vi "调阀对中 对中偏振角度.vi"(9 "角度":dbl[](array[numeric]), 10 "油压":dbl[](array[numeric]), 11 "扭矩":dbl[](array[numeric])) -> (1 "偏差角度":dbl, 3 "偏差扭矩":dbl format="%0.2f")   [LabVIEW 2015, in "Logging.lvlib"]
uses:
  Logging.lvlib
  <vilib>/Analysis/1siggen.llb/Ramp Pattern by Samples.vi
  <vilib>/Analysis/baseanly.llb/Mean (DBL).vi
  <vilib>/gmath/NI_Gmath.lvlib
  <vilib>/Analysis/NI_AALBase.lvlib
panel:
  out "角度反转回":dbl[](array[numeric])
  out "角度反转去":dbl[](array[numeric])
  out "角度正转回":dbl[](array[numeric])
  out "角度正转去":dbl[](array[numeric])
  out "油压反转回":dbl[](array[numeric])
  out "油压反转去":dbl[](array[numeric])
  out "油压正转回":dbl[](array[numeric])
  out "油压正转去":dbl[](array[numeric])
  out "扭矩反转回":dbl[](array[numeric])
  out "扭矩反转去":dbl[](array[numeric])
  out "扭矩正转回":dbl[](array[numeric])
  out "扭矩正转去":dbl[](array[numeric])
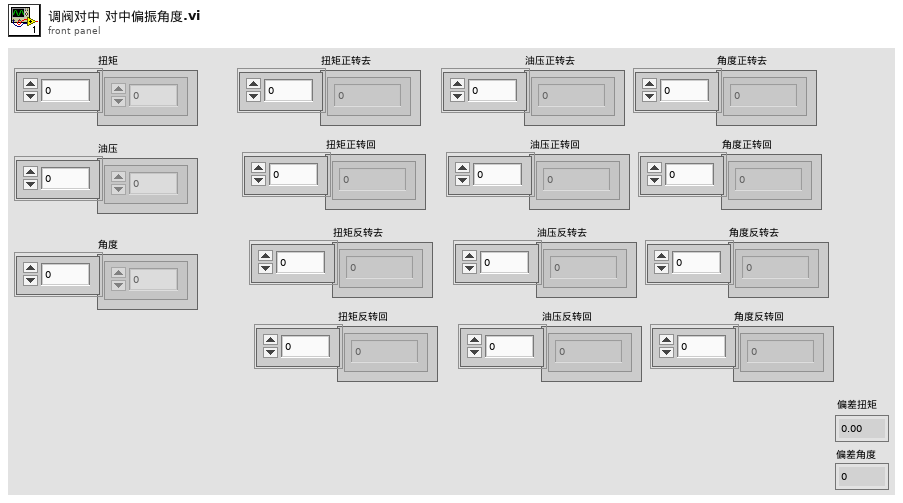
[diagram p1: front panel]
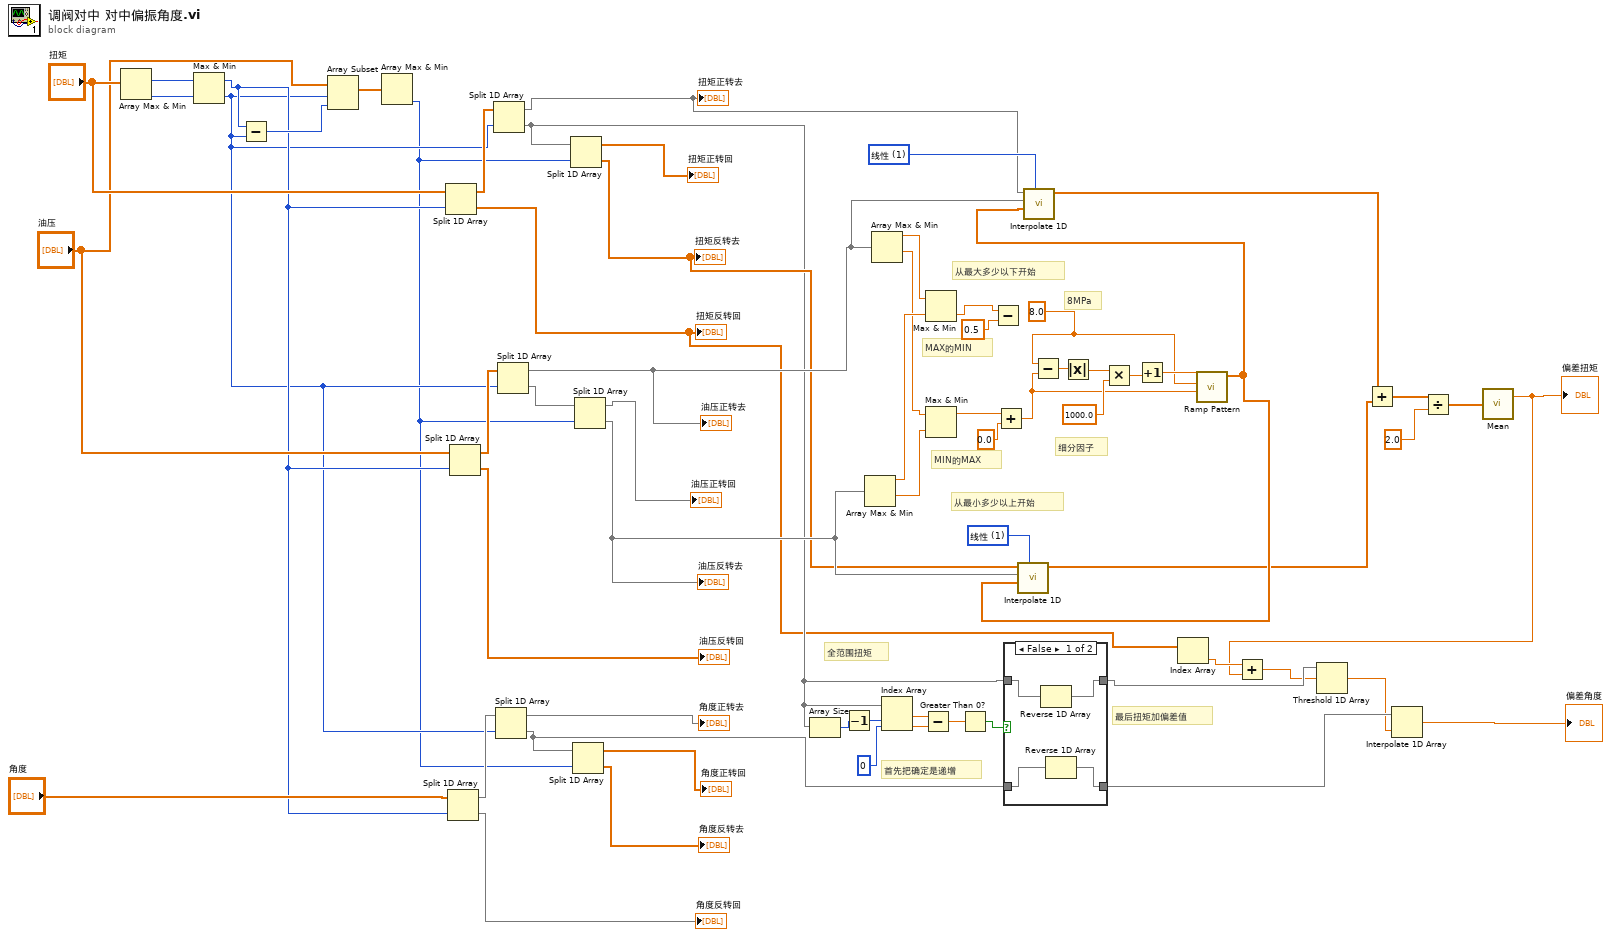
[diagram p0: block diagram]
diagram:
  w32 = 8.0 ("x")
  w35 = 1 items=["最近", "线性", "样条", "cubic Hermite", "拉格朗日"] ("method")
  w48 = 1 items=["最近", "线性", "样条", "cubic Hermite", "拉格朗日"] ("method")
  # "最后扭矩加偏差值"
  # "首先把确定是递增"
  # "全范围扭矩"
  # "8MPa"
  # "细分因子"
  # "从最大多少以下开始"
  # "从最小多少以上开始"
  # "MIN的MAX"
  # "MAX的MIN"
  n1 = Array Max & Min(array="扭矩") -> (max index (indices)=w65:i32, min index (indices)=w64:i32)  [unwired: 2 out]
  n2 = Max & Min(x=w65, y=w64) -> (max(x,y)=w51:i32, min(x,y)=w50:i32)
  n3 = Subtract(x=w51, y=w50) -> (x-y=w61:i32)
  n4 = Array Subset(array="油压", index=w50, length=w61) -> (w60:dbl[])
  n5 = Array Max & Min(array=w60) -> (min index (indices)=w49:i32)  [unwired: 3 out]
  n6 = Split 1D Array(array="扭矩", index=w51) -> (first subarray=w62:dbl[], second subarray=w7:dbl[])
  "扭矩反转回" <- w7
  n7 = Split 1D Array(array="角度", index=w51) -> (first subarray=w53:dbl[], second subarray=→"角度反转回":dbl[])
  n8 = Split 1D Array(array="油压", index=w51) -> (first subarray=w58:dbl[], second subarray=→"油压反转回":dbl[])
  n9 = Split 1D Array(array=w62, index=w50) -> (first subarray=w19:dbl[], second subarray=w10:dbl[])
  "扭矩正转去" <- w19
  n10 = Split 1D Array(array=w53, index=w50) -> (first subarray=→"角度正转去":dbl[], second subarray=w9:dbl[])
  n11 = Split 1D Array(array=w58, index=w50) -> (first subarray=w30:dbl[], second subarray=w57:dbl[])
  "油压正转去" <- w30
  n12 = Split 1D Array(array=w10, index=w49) -> (first subarray=→"扭矩正转回":dbl[], second subarray=w18:dbl[])
  "扭矩反转去" <- w18
  n13 = Split 1D Array(array=w9, index=w49) -> (first subarray=→"角度正转回":dbl[], second subarray=→"角度反转去":dbl[])
  n14 = Split 1D Array(array=w57, index=w49) -> (first subarray=→"油压正转回":dbl[], second subarray=w26:dbl[])
  "油压反转去" <- w26
  n15 = Array Size(array=w10) -> (size(s)=w15:i32)
  n16 = Decrement(x=w15) -> (x-1=w16:i32)
  n17 = Array Max & Min(array=w26) -> (max value=w46:dbl, min value=w44:dbl)  [unwired: 2 out]
  n18 = Array Max & Min(array=w30) -> (max value=w47:dbl, min value=w45:dbl)  [unwired: 2 out]
  n19 = Index Array(array=w10, index #1=w16, index #2=0 ("索引")) -> (element #1=w13:dbl, element #2=w14:dbl)
  n20 = Subtract(x=w13, y=w14) -> (x-y=w12:dbl)
  n21 = Max & Min(x=w47, y=w46) -> (min(x,y)=w33:dbl)  [unwired: 1 out]
  n22 = Max & Min(x=w45, y=w44) -> (max(x,y)=w34:dbl)  [unwired: 1 out]
  n23 = Greater Than 0?(x=w12) -> (x > 0?=w11:bool)
  n24 = Subtract(x=w33, y=0.5) -> ()  [unwired: 1 out]
  n25 = Add(x=w34, y=0.0) -> (x+y=w36:dbl)
  n26 = case shown="False" w11 {
    tunnel: w10 -> [w69 w71]
    tunnel: [w68 w71] -> w5
    tunnel: w9 -> [w67 w70]
    tunnel: [w66 w70] -> w3
    frame False {
      n27 = Reverse 1D Array(array=w69) -> (reversed array=w68:dbl[])
      n28 = Reverse 1D Array(array=w67) -> (reversed array=w66:dbl[])
    }
    frame True {
      # "递增"
    }
  }
  n29 = Subtract(x=w32, y=w36) -> (x-y=w41:dbl)
  n30 = Absolute Value(x=w41) -> (abs(x)=w39:dbl)
  n31 = Multiply(x=w39, y=1000.0) -> (x*y=w40:dbl)
  n32 = Increment(x=w40) -> (x+1=w37:dbl)
  n33 = Index Array(array=w7) -> (element=w8:dbl)  [unwired: 1 in]
  n34 = call-poly <vilib>:"Ramp Pattern.vi"("start"=w36, "end"=w32, "samples"=w37) -> ("Ramp Pattern"=w31:dbl[])  [unwired: 7 in, 1 out]
  n35 = call <vilib>:"Interpolate 1D.vi"("method"=w35, "xi"=w31, "X"=w26, "Y"=w18) -> ("yi"=w23:dbl[])  [unwired: 5 in, 2 out]
  n36 = call <vilib>:"Interpolate 1D.vi"("method"=w48, "xi"=w31, "X"=w30, "Y"=w19) -> ("yi"=w24:dbl[])  [unwired: 5 in, 2 out]
  n37 = Add(x=w24, y=w23) -> (x+y=w21:dbl[])
  n38 = Divide(x=w21, y=2.0) -> (x/y=w20:dbl[])
  n39 = call-poly <vilib>:"Mean.vi"("X"=w20) -> ("mean"=w6:dbl)  [unwired: 1 out]
  "偏差扭矩" <- w6
  n40 = Add(x=w8, y=w6) -> (x+y=w4:dbl)
  n41 = Threshold 1D Array(2:w4, 3:w5) -> (0:w2:dbl)  [unwired: 1 in]
  n42 = Interpolate 1D Array(1:w2, 2:w3) -> (0:→"偏差角度":dbl)
